vi "DB Tools Build Select Query.vi"(5 "columns":string[](array[string]), 6 "table name":string) -> (3 "select query":string)   [LabVIEW 2012, in "NI_Database_API_64.lvlib"]
doc: "Creates the SQL SELECT query string based on the table and column information provided."
uses:
  NI_Database_API_64.lvlib
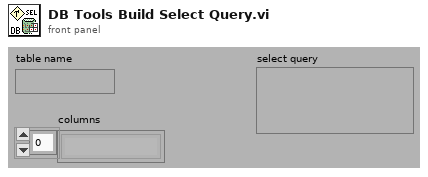
[diagram p1: front panel]
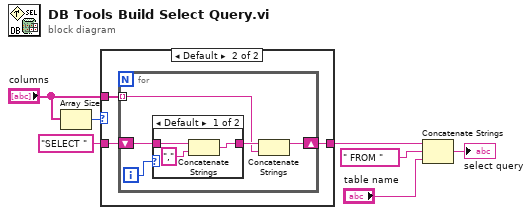
[diagram p0: block diagram]
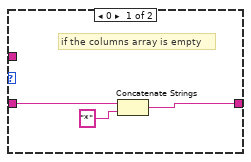
[diagram p2: hidden frame]
diagram:
  n1 = Array Size(array="columns") -> (size(s)=w7:i32)
  n2 = case shown="Default" w7 {
    tunnel: "columns" -> [_ w13]
    tunnel: [w9 w12] -> w5
    tunnel: "SELECT " ("Substring") -> [w8 w11]
    frame 0 {
      # "if the columns array is empty"
      n3 = Concatenate Strings(w8, "*" ("Substring")) -> (w9:string)
    }
    frame Default {
      n4 = for {
        tunnel: w13 -> [w15] mode=indexing
        shift-right: [w14] -> w12
        shift-left: w11 -> [w17]
        i -> [w18]
        n5 = case shown="Default" w18 {
          tunnel: w17 -> [w21 w22]
          tunnel: [w19 w22] -> w16
          frame Default {
            n6 = Concatenate Strings(w21, "," ("Substring")) -> (w19:string)
          }
          frame 0 {
          }
        }
        n7 = Concatenate Strings(w16, w15) -> (w14:string)
      }
    }
  }
  n8 = Concatenate Strings(w5, " FROM " ("Substring"), "table name") -> (→"select query":string)
